vi "TestVI.vi"() -> ()   [LabVIEW 2016]
uses:
  DAQcamera.lvclass
  C:/Users/curtis.gutjahr/Documents/Labview Code/CTControl Code/PI Utilities/DAQclass/DAQdevice/DAQdevice.lvclass
  DAQdevice/DAQdevice.lvclass
  DAQcamera.lvclass/DAQcamera.ctl
panel:
  out "cam arm error":errorcluster
  out "Array":errorcluster[](array[cluster])
  in  "Camera SN U64":u64
  in  "error in":errorcluster
  in  "DAQcamera.lvclass":refnum<class "DAQcamera.lvclass">
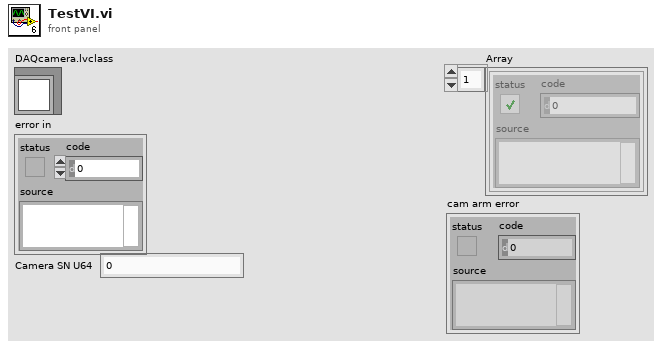
[diagram p1: front panel]
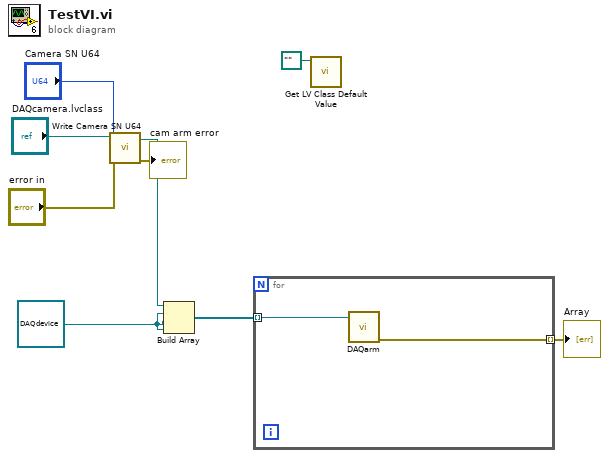
[diagram p0: block diagram]
diagram:
  w6 = refnum<class "DAQdevice.lvclass"> refnum ("DAQdevice.lvclass")
  n1 = call "Write Camera SN U64.vi"("error in (no error)"="error in", "Camera SN U64"="Camera SN U64", "DAQcamera in"="DAQcamera.lvclass") -> ("error out"=→"cam arm error":errorcluster, "DAQcamera out"=w7:refnum<class "DAQcamera.lvclass">)  [unwired: 7 in]
  n2 = Build Array(w7, w6, w6, w6) -> (w5:refnum<class "DAQdevice.lvclass">[])
  n3 = for {
    tunnel: w5 -> [w11] mode=indexing
    tunnel: [w10] -> w4 mode=indexing
    n4 = call-dynamic "DAQarm.vi"("DAQdevice in"=w11) -> ("error out"=w10:errorcluster)  [unwired: 9 in, 1 out]
  }
  "Array" <- w4
  n5 = call <vilib>:"Get LV Class Default Value.vi"("class path"=path "") -> ()  [unwired: 9 in, 2 out]
